vi "Get Table Time datatype.vi"(8 "error in (no error)":errorcluster, 10 "Table path":string, 11 "LV-Data.PGSQL in":refnum<class "LV-Data.PGSQL.lvclass">) -> (0 "error out":errorcluster, 2 "Time Datatype":T1, 3 "LV-Data.PGSQL out":refnum<class "LV-Data.PGSQL.lvclass">)   [LabVIEW 2019, in "LV-Data.PGSQL.lvclass"]
uses:
  LV-Data.PGSQL.lvclass
  Typedefs/Time.Datatype--enum.ctl
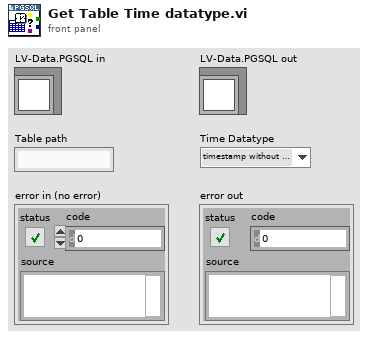
[diagram p1: front panel]
types:
  T1 = typedef "LV-Data.PGSQL.lvclass/Time.Datatype--enum.ctl" = enum16{"timestamp without time zone", "timestamp with time zone"}
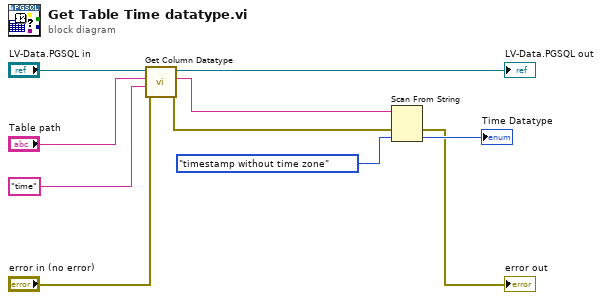
[diagram p0: block diagram]
diagram:
  n1 = call "Get Column Datatype.vi"("error in (no error)"="error in (no error)", "Column Name"="time", "Table Path"="Table path", "LV-Data.PGSQL in"="LV-Data.PGSQL in") -> ("error out"=w4:errorcluster, "Datatype"=w1:string, "LV-Data.PGSQL out"=→"LV-Data.PGSQL out":refnum<class "LV-Data.PGSQL.lvclass">)  [unwired: 5 in]
  n2 = Scan From String(input string=w1, error in=w4, default 1=Time.Datatype--enum."timestamp without time zone" ("Time Datatype")) -> (error out=→"error out":errorcluster, output 1=→"Time Datatype":T1)  [unwired: 2 in, 2 out]
